vi "getTrackControls.vi"(7 "LabVIEW Web Service Request":refnum<class "Web Request.lvclass">) -> ()   [LabVIEW 2014]
uses:
  <vilib>/wsapi/Web Request.lvclass
  Controls/Track Controls.ctl
  Controls/Track Volume Settings.ctl
panel:
  in  "Track Controls":T1 {"Track 3"."Volume" scale=0.01..10.0; "Track 3"."Pan" scale=0.0..1.0; "Track 2"."Volume" scale=0.01..10.0; "Track 2"."Pan" scale=0.0..1.0; "Track 1"."Volume" scale=0.01..10.0; "Track 1"."Pan" scale=0.0..1.0; "Track 0"."Volume" scale=0.01..10.0; "Track 0"."Pan" scale=0.0..1.0}
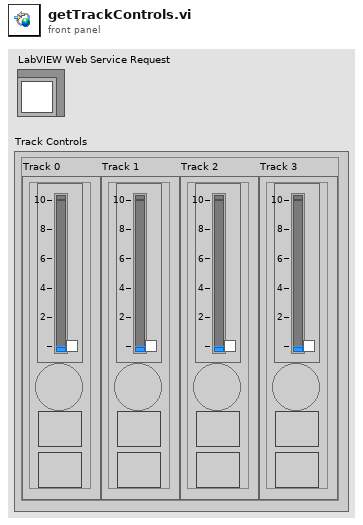
[diagram p1: front panel]
types:
  T1 = typedef "Track Controls.ctl" = cluster{"Track 0":T2, "Track 1":T2, "Track 2":T2, "Track 3":T2}
  T2 = typedef "Track Volume Settings.ctl" = cluster{"Volume":dbl, "Pan":dbl, "Record":bool, "FX":bool}
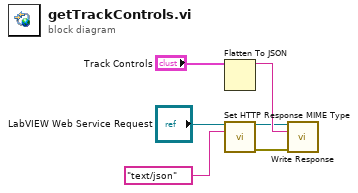
[diagram p0: block diagram]
diagram:
  n1 = Flatten To JSON(anything="Track Controls") -> (JSON string=w6:string)  [unwired: 2 in, 1 out]
  n2 = call <vilib>:"Set HTTP Response MIME Type.vi"("LabVIEW Web Service Request"="LabVIEW Web Service Request", "MIME type (text/html)"="text/json") -> ("LabVIEW Web Service Request out"=w5:refnum<class "Web Request.lvclass">, "error out"=w4:errorcluster)  [unwired: 12 in]
  n3 = call <vilib>:"Write Response.vi"("LabVIEW Web Service Request"=w5, "response string"=w6, "error in (no error)"=w4) -> ()  [unwired: 11 in, 2 out]
